vi "Read VI Refnum.vi"(8 "error in (no error)":errorcluster, 11 "Panel in":refnum<class "Panel.lvclass">) -> (0 "error out":errorcluster, 2 "VI Refnum":refnum<vi>)   [LabVIEW 2023, in "Panel Actor.lvlib" / "Panel.lvlib" / "Panel.lvclass"]
doc: "Reads the current panel's VI refnum.\n----\nCopyright: MGI 2016\nAuthor: Derek Trepanier"
uses:
  Panel.lvclass
  Panel.lvclass/Panel.ctl
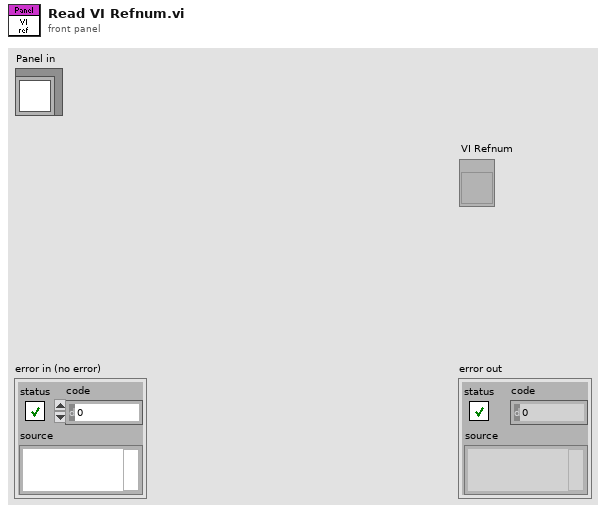
[diagram p1: front panel]
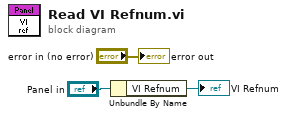
[diagram p0: block diagram]
diagram:
  n1 = Unbundle By Name("Panel in") -> ("VI Refnum"=→"VI Refnum":refnum<vi>)
  "error out" <- "error in (no error)"
